vi "GetUIState.vi"(6 "timeout in ms (-1)":i32, 8 "error in (no error)":errorcluster, 11 "EmbeddedSMO in":refnum<class "Embedded UI.lvclass">) -> (0 "error out":errorcluster, 2 "UI State":T1=enum."Embedded", 3 "EmbeddedSMO out":refnum<class "Embedded UI.lvclass">)   [LabVIEW 2019, in "Embedded UI.lvclass"]
uses:
  Embedded UI.lvclass
  Typedefs/UI State.ctl
  Typedefs/PrivateEvents--Embedded UI.Get UI State.ctl
  Typedefs/GetUIStateNotifier.ctl
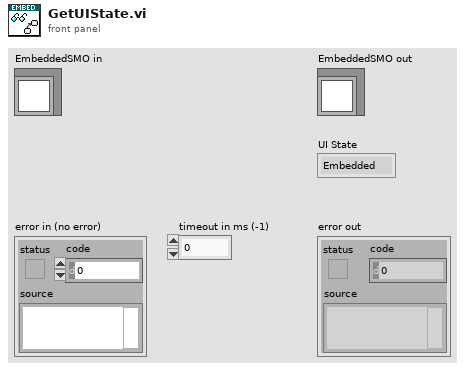
[diagram p1: front panel]
types:
  T1 = typedef "Embedded UI.lvclass/UI State.ctl" = enum16{"unknown", "Opened", "Embedded", "Closed"}
  T2 = typedef "Embedded UI.lvclass/PrivateEvents--Embedded UI.Get UI State.ctl" = cluster{"Notifier":T3}
  T3 = typedef "Embedded UI.lvclass/GetUIStateNotifier.ctl" = refnum<notifier>
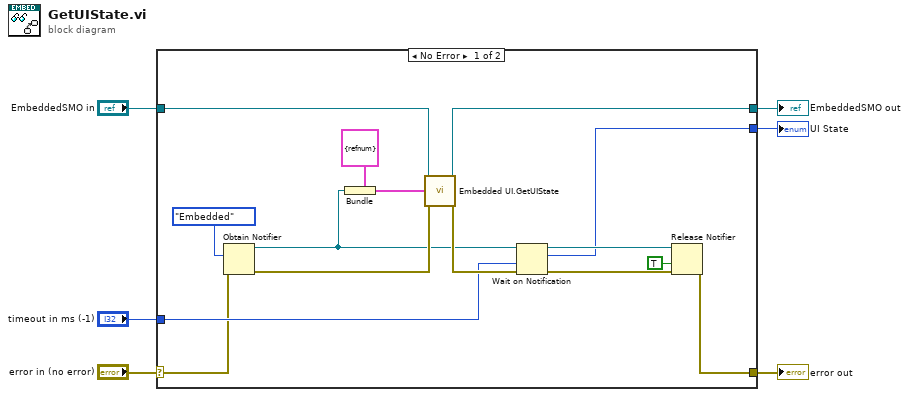
[diagram p0: block diagram]
diagram:
  n1 = case shown="No Error" "error in (no error)" {
    selector: "error in (no error)" -> [w8 w23]
    tunnel: [w7 w23] -> w5
    tunnel: [w9 w22] -> w3
    tunnel: "EmbeddedSMO in" -> [w10 w22]
    tunnel: [w12 _] -> w2
    tunnel: "timeout in ms (-1)" -> [w11 _]
    frame No Error {
      n2 = Obtain Notifier(notification data type=UI_State."Embedded" ("UI State 2"), error in (no error)=w8) -> (notifier out=w16:refnum<notifier>, error out=w18:errorcluster)  [unwired: 2 in, 1 out]
      n3 = Bundle(cluster=T2 {"Notifier"=refnum} ("Get UI State"), "Notifier"=w16) -> (w21:T2)
      n4 = call "Embedded UI.GetUIState.vi"("error in (no error)"=w18, "Get UI State"=w21, "EmbeddedSMO"=w10) -> ("error out"=w17:errorcluster, "EmbeddedSMO out"=w9:refnum<class "Embedded UI.lvclass">)  [unwired: 7 in]
      n5 = Wait on Notification(notifier=w16, timeout in ms (-1)=w11, error in (no error)=w17) -> (notifier out=w15:refnum<notifier>, notification=w12:T1, error out=w13:errorcluster)  [unwired: 1 in, 1 out]
      n6 = Release Notifier(notifier=w15, force destroy? (F)=TRUE, error in (no error)=w13) -> (error out=w7:errorcluster)  [unwired: 2 out]
    }
    frame Error {
    }
  }
  "error out" <- w5
  "EmbeddedSMO out" <- w3
  "UI State" <- w2
